vi "GetClusterReference.vi"(8 "error in":errorcluster, 11 "Cluster in":refnum<class "Cluster.lvclass">) -> (0 "error out":errorcluster, 1 "cluster reference":refnum<vi>, 3 "Cluster out":refnum<class "Cluster.lvclass">)   [LabVIEW 2014, in "Cluster.lvclass"]
uses:
  Cluster.lvclass
  Generic/Generic.lvclass
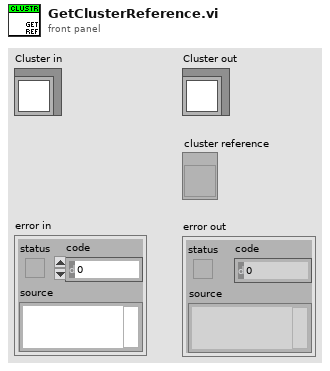
[diagram p1: front panel]
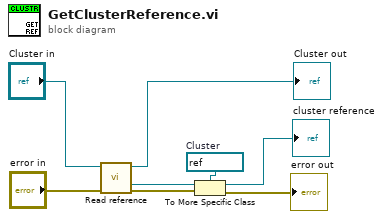
[diagram p0: block diagram]
diagram:
  w2 = refnum<vi> refnum  # Cluster
  n1 = call "Read reference.vi"("error in"="error in", "GObject in"="Cluster in") -> ("error out"=w6:errorcluster, "reference"=w5:refnum<vi>, "GObject out"=→"Cluster out":refnum<class "Cluster.lvclass">)  [unwired: 5 in]
  n2 = To More Specific Class(target class=w2, reference=w5, error in=w6) -> (specific class reference=→"cluster reference":refnum<vi>, error out=→"error out":errorcluster)
